vi "LEDbegin.vi"   [LabVIEW 2015]
uses:
  <vilib>/Rock Robotics/SystemInterfaces/DIO/FPGA_DIOChannel.ctl
  <vilib>/Rock Robotics/WPI/AnalogOutput/WPI_AnalogOutputChannel.ctl
types:
  T1 = typedef "FPGA_DIOChannel.ctl" = enum8{"DIO 0", "DIO 1", "DIO 2", "DIO 3", "DIO 4", "DIO 5", "DIO 6", "DIO 7", "DIO 8", "DIO 9", "DIO MXP 0", "DIO MXP 1", "DIO MXP 2", "DIO MXP 3", "DIO MXP 4", "DIO MXP 5", "DIO MXP 6", "DIO MXP 7", "DIO MXP 8", "DIO MXP 9", "DIO MXP 10", "DIO MXP 11", "DIO MXP 12", "DIO MXP 13", "DIO MXP 14", "DIO MXP 15", "Invalid"}
  T2 = typedef "WPI_AnalogOutputChannel.ctl" = enum8{"AO MXP 0", "AO MXP 1", "Invalid"}
  T3 = typedef "WPI_AOChannelDevRef.ctl" = cluster{"DevStatus":errorcluster, "AO Channel":T2}
  T4 = typedef "WPI_DigitalOutputDevRef.ctl" = cluster{"DIO Channel":T1, "DevStatus":errorcluster}
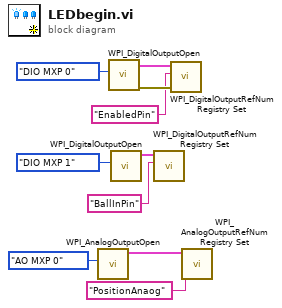
[diagram p0: block diagram]
diagram:
  n1 = call <vilib>:"WPI_AnalogOutputOpen.vi"("AO Channel"=WPI_AnalogOutputChannel."AO MXP 0") -> ("AODeviceRef"=w5:T3)  [unwired: 9 in, 1 out]
  n2 = call <vilib>:"WPI_DigitalOutputOpen.vi"("DIO Channel"=FPGA_DIOChannel."DIO MXP 0") -> ("error out"=w10:errorcluster, "DigitalOutputDevRef"=w9:T4)  [unwired: 9 in]
  n3 = call <vilib>:"WPI_DigitalOutputOpen.vi"("DIO Channel"=FPGA_DIOChannel."DIO MXP 1") -> ("DigitalOutputDevRef"=w3:T4)  [unwired: 9 in, 1 out]
  n4 = call <vilib>:"WPI_DigitalOutputRefNum Registry Set.vi"("refnum name"="BallInPin", "DigitalOutputDevRef"=w3) -> ()  [unwired: 8 in, 2 out]
  n5 = call <vilib>:"WPI_DigitalOutputRefNum Registry Set.vi"("error in (no error)"=w10, "refnum name"="EnabledPin", "DigitalOutputDevRef"=w9) -> ()  [unwired: 7 in, 2 out]
  n6 = call <vilib>:"WPI_AnalogOutputRefNum Registry Set.vi"("refnum name"="PositionAnaog", "AODeviceRef"=w5) -> ()  [unwired: 8 in, 2 out]
